vi "13.-Dar Formato a un Archivo de Lectura de Datos.vi"() -> ()   [LabVIEW 2017]
panel:
  out "error out":errorcluster
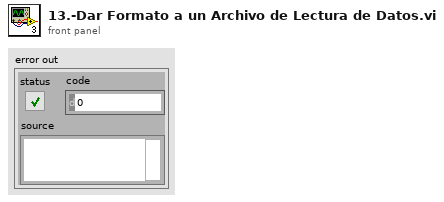
[diagram p1: front panel]
types:
  T1 = enum16{"open", "replace", "create", "open or create", "replace or create", "replace or create with confirmation"}
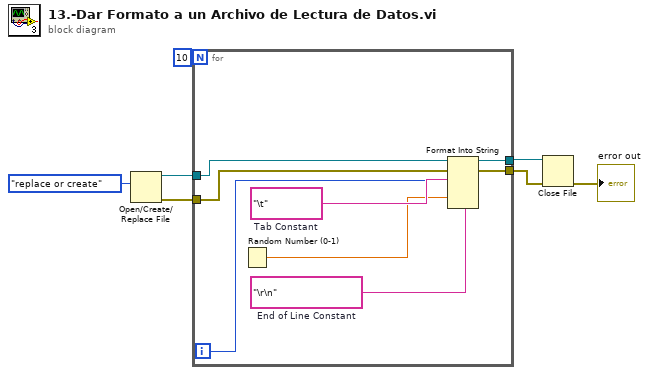
[diagram p0: block diagram]
diagram:
  n1 = Open/Create/Replace File(operation (0:open)=T1."replace or create") -> (refnum out=w5:refnum<file>, error out=w4:errorcluster)  [unwired: 5 in, 1 out]
  n2 = for {
    N: 10 -> [_]
    tunnel: w5 -> [w15]
    tunnel: w4 -> [w14]
    tunnel: [w13] -> w3
    tunnel: [w12] -> w2
    i -> [w9]
    w8 = "\r\n"  # End of Line Constant
    w11 = "\t"  # Tab Constant
    n3 = Random Number (0-1)() -> (number: 0 to 1=w10:dbl)
    n4 = Format Into String(initial string=w15, error in=w14, w9, w11, w10, w8) -> (resulting string=w13:refnum<file>, error out=w12:errorcluster)  [unwired: 1 in]
  }
  n5 = Close File(refnum=w3, error in=w2) -> (error out=→"error out":errorcluster)  [unwired: 1 out]
